vi "exert.vi"(11 "Boolean":bool) -> ()   [LabVIEW 2015]
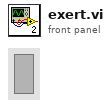
[diagram p1: front panel]
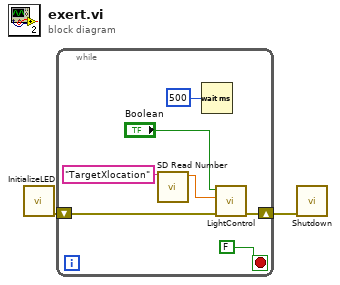
[diagram p0: block diagram]
diagram:
  n1 = call "InitializeLED.vi"() -> ("error out"=w2:errorcluster)  [unwired: 11 in]
  n2 = while {
    shift-right: [w6] -> w1
    shift-left: w2 -> [w9]
    stop <- FALSE ("stop") stop-if-true
    n3 = call <vilib>:"SD Read Number.vi"("Name"="TargetXlocation") -> ("Numeric"=w4:dbl)  [unwired: 8 in, 2 out]
    n4 = Wait (ms)(milliseconds to wait=u32 500) -> ()  [unwired: 1 out]
    n5 = call "LightControl.vi"("error in (no error)"=w9, "X"=w4, "Boolean"="Boolean") -> ("error out"=w6:errorcluster)  [unwired: 8 in]
  }
  n6 = call "Shutdown.vi"("error in (no error)"=w1) -> ()  [unwired: 10 in, 1 out]
